vi "Get Pi Data.vi"(8 "error in (no error)":errorcluster, 11 "connection ID":refnum<k16>) -> (0 "error out":errorcluster, 3 "values":T1)   [LabVIEW 2016]
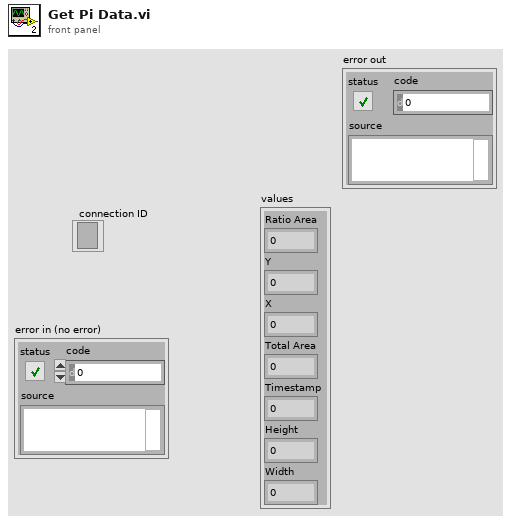
[diagram p1: front panel]
types:
  T1 = cluster{"Ratio Area":dbl, "Y":dbl, "X":dbl, "Total Area":dbl, "Timestamp":ext, "Height":dbl, "Width":dbl}
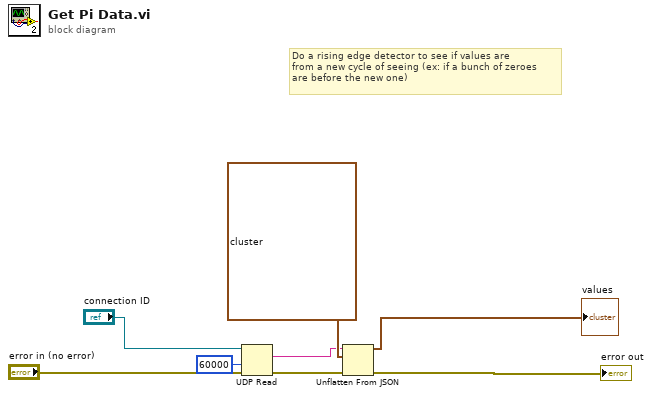
[diagram p0: block diagram]
diagram:
  # "Do a rising edge detector to see if values are \nfrom a new cycle of seeing (ex: if a bunch of zeroes\nare before the new one)"
  n1 = UDP Read(connection ID="connection ID", timeout ms (25000)=60000, 8:"error in (no error)") -> (data out=w5:string, error out=w4:errorcluster)  [unwired: 1 in, 3 out]
  n2 = Unflatten From JSON(JSON string=w5, type and defaults=T1 {"Ratio Area"=0.0, "Y"=0.0, "X"=0.0, "Total Area"=0.0, "Timestamp"=0.0, "Height"=0.0, "Width"=0.0}, error in (no error)=w4) -> (value=→"values":T1, error out=→"error out":errorcluster)  [unwired: 4 in]
